vi "Vision Processing.vi"(4 "error in (no error)":errorcluster, 7 "Image Size":T1=enum."320x240") -> ()   [LabVIEW 2015]
doc: "This VI runs in parallel to other tasks. It gets images from the camera, processes them for color or shape and use that information to affect robot behavior."
uses:
  Robot Global Data.vi
  <vilib>/Rock Robotics/WPI/Camera/WPI_CameraWhite Balance Values.ctl
  <vilib>/Rock Robotics/WPI/Camera/WPI_CameraExposure Values.ctl
  <vilib>/Rock Robotics/WPI/Camera/WPI_CameraFrameRate.ctl
  <vilib>/Rock Robotics/WPI/Camera/WPI_CameraImageSize.ctl
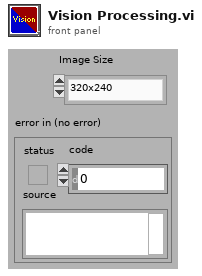
[diagram p1: front panel]
types:
  T1 = typedef "WPI_CameraImageSize.ctl" = enum16{"640x480", "320x240", "160x120"}
  T2 = typedef "WPI_CameraFrameRate.ctl" = u32
  T3 = typedef "WPI_CameraExposure Values.ctl" = enum16{"Auto", "Flicker-free 50 Hz", "Flicker-free 60 Hz", "Hold current"}
  T4 = typedef "WPI_CameraWhite Balance Values.ctl" = enum16{"Auto", "Fixed indoor", "Fixed outdoor 1", "Fixed outdoor 2", "Fixed fluorescent 1", "Fixed fluorescent 2", "Hold current"}
  T5 = typedef "Image Type" = u32
  T6 = typedef "WPI_CameraDevRef.ctl" = cluster{"Camera Address":string, "CameraStatus":errorcluster, "Acquire Image Notifier":refnum<notifier>}
  T7 = typedef "IMAQ Image.ctl" = refnum<image>
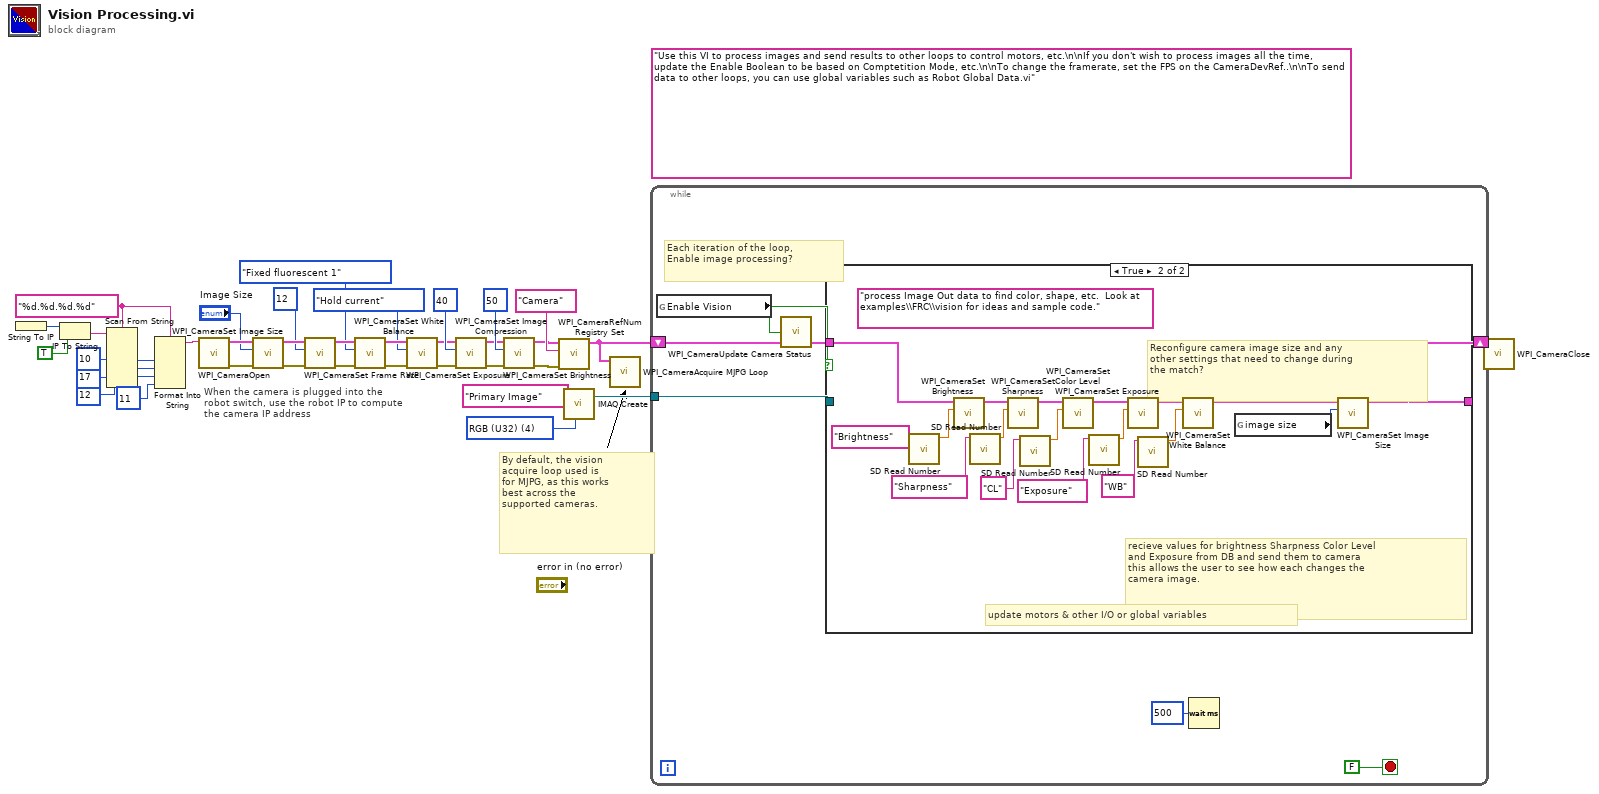
[diagram p0: block diagram]
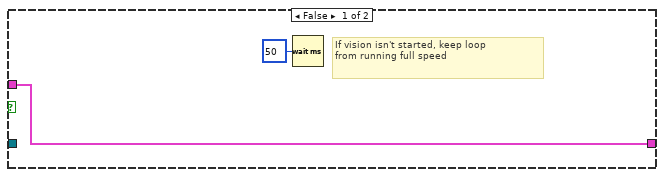
[diagram p2: hidden frame]
diagram:
  w8 = "%d.%d.%d.%d" ("format string")
  (unwired) "Use this VI to process images and send results to other loops to control motors, etc.\n\nIf you don't wish to process images all the time, update the Enable Boolean to be based on Comptetition Mode, etc.\n\nTo change the framerate, set the FPS on the CameraDevRef..\n\nTo send data to other loops, you can use global variables such as Robot Global Data.vi"
  w38 = T5 4 items=["Grayscale (U8)", "Grayscale (I16)", "Grayscale (SGL)", "Complex (CSG)", "RGB (U32)", "HSL (U32)", "RGB (U64)"] ("Image Type")
  # "When the camera is plugged into the\nrobot switch, use the robot IP to compute\nthe camera IP address"
  # "By default, the vision\nacquire loop used is\nfor MJPG, as this works\nbest across the\nsupported cameras."
  n1 = String To IP() -> (0:w15:u32)  [unwired: 1 in]
  n2 = IP To String(1:TRUE ("dot notation? (F)"), 2:w15) -> (0:w13:string)
  n3 = Scan From String(format string=w8, input string=w13, default 1=10 ("default value 1"), default 2=17 ("default value 2"), default 3=12 ("default value 3")) -> (output 1=w12:i32, output 2=w11:i32, output 3=w10:i32)  [unwired: 4 in, 3 out]
  n4 = Format Into String(format string=w8, w12, w11, w10, 11 ("Compression")) -> (resulting string=w7:string)  [unwired: 2 in, 1 out]
  n5 = call <vilib>:"WPI_CameraOpen.vi"("Camera Address"=w7) -> ("error out"=w26:errorcluster, "CameraDevRef"=w27:T6)  [unwired: 1 in, 8 out]
  n6 = call <vilib>:"WPI_CameraSet Image Size.vi"("error in (no error)"=w26, "Image Size"="Image Size", "CameraDevRef"=w27) -> ("error out"=w25:errorcluster, "CameraDevRef Out"=w28:T6)  [unwired: 7 out]
  n7 = call <vilib>:"WPI_CameraSet Frame Rate.vi"("error in (no error)"=w25, "Frame Rate (fps)"=T2 12, "CameraDevRef"=w28) -> ("error out"=w24:errorcluster, "CameraDevRef Out"=w30:T6)  [unwired: 7 out]
  n8 = call <vilib>:"WPI_CameraSet White Balance.vi"("error in (no error)"=w24, "White Balance"=WPI_CameraWhite_Balance_Values."Fixed fluorescent 1", "CameraDevRef"=w30) -> ("error out"=w23:errorcluster, "CameraDevRef Out"=w29:T6)  [unwired: 7 out]
  n9 = call <vilib>:"WPI_CameraSet Exposure.vi"("error in (no error)"=w23, "Exposure"=WPI_CameraExposure_Values."Hold current", "CameraDevRef"=w29) -> ("error out"=w22:errorcluster, "CameraDevRef Out"=w32:T6)  [unwired: 7 out]
  n10 = call <vilib>:"WPI_CameraSet Image Compression.vi"("error in (no error)"=w22, "Compression"=40, "CameraDevRef"=w32) -> ("error out"=w21:errorcluster, "CameraDevRef Out"=w31:T6)  [unwired: 7 out]
  n11 = call <vilib>:"WPI_CameraSet Brightness.vi"("error in (no error)"=w21, "Brightness"=50, "CameraDevRef"=w31) -> ("error out"=w19:errorcluster, "CameraDevRef Out"=w20:T6)  [unwired: 7 out]
  n12 = call <vilib>:"WPI_CameraRefNum Registry Set.vi"("error in (no error)"=w19, "refnum name"="Camera", "CameraDevRef"=w20) -> ("CameraDevRef"=w6:T6)  [unwired: 8 out]
  n13 = call "IMAQ Create"("Image Name"="Primary Image", "Image Type"=w38) -> ("New Image"=w36:T7)  [unwired: 2 in, 2 out]
  n14 = call <vilib>:"WPI_CameraAcquire MJPG Loop.vi"("CameraDevRef"=w6) -> ()  [unwired: 11 in]
  n15 = while {
    shift-right: [w42] -> w4
    shift-left: w6 -> [w45]
    tunnel: w36 -> [w44]
    stop <- FALSE stop-if-true
    # "Each iteration of the loop,\nEnable image processing?"
    n16 = global read "Robot Global Data.vi" "Enable Vision"() -> (w43:bool)
    n17 = call <vilib>:"WPI_CameraUpdate Camera Status.vi"("CameraDevRef In"=w45, "Enable Vision"=w43) -> ("CameraDevRef Out"=w41:T6)  [unwired: 3 in]
    n18 = case shown="True" w43 {
      tunnel: [w46 w65] -> w42
      tunnel: w44 -> [_ _]
      tunnel: w41 -> [w46 w48]
      frame False {
        # "If vision isn't started, keep loop\nfrom running full speed"
        n19 = Wait (ms)(milliseconds to wait=u32 50) -> ()  [unwired: 1 out]
      }
      frame True {
        (unwired) "process Image Out data to find color, shape, etc.  Look at examples\\FRC\\vision for ideas and sample code."
        # "recieve values for brightness Sharpness Color Level\nand Exposure from DB and send them to camera\nthis allows the user to see how each changes the \ncamera image."
        # "update motors & other I/O or global variables"
        # "Reconfigure camera image size and any\nother settings that need to change during\nthe match?"
        n20 = call <vilib>:"SD Read Number.vi"("Name"="Brightness") -> ("Numeric"=w60:dbl)  [unwired: 8 in, 2 out]
        n21 = call <vilib>:"WPI_CameraSet Brightness.vi"("Brightness"=w60, "CameraDevRef"=w48) -> ("CameraDevRef Out"=w62:T6)  [unwired: 8 in, 1 out]
        n22 = call <vilib>:"SD Read Number.vi"("Name"="Sharpness") -> ("Numeric"=w54:dbl)  [unwired: 8 in, 2 out]
        n23 = call <vilib>:"WPI_CameraSet Sharpness.vi"("Sharpness"=w54, "CameraDevRef"=w62) -> ("CameraDevRef Out"=w63:T6)  [unwired: 8 in, 1 out]
        n24 = call <vilib>:"SD Read Number.vi"("Name"="CL") -> ("Numeric"=w53:dbl)  [unwired: 8 in, 2 out]
        n25 = call <vilib>:"WPI_CameraSet Color Level.vi"("Color Level"=w53, "CameraDevRef"=w63) -> ("CameraDevRef Out"=w61:T6)  [unwired: 8 in, 1 out]
        n26 = call <vilib>:"SD Read Number.vi"("Name"="Exposure") -> ("Numeric"=w56:dbl)  [unwired: 8 in, 2 out]
        n27 = call <vilib>:"WPI_CameraSet Exposure.vi"("Exposure"=w56, "CameraDevRef"=w61) -> ("CameraDevRef Out"=w52:T6)  [unwired: 8 in, 1 out]
        n28 = call <vilib>:"SD Read Number.vi"("Name"="WB") -> ("Numeric"=w50:dbl)  [unwired: 8 in, 2 out]
        n29 = call <vilib>:"WPI_CameraSet White Balance.vi"("White Balance"=w50, "CameraDevRef"=w52) -> ("CameraDevRef Out"=w51:T6)  [unwired: 8 in, 1 out]
        n30 = global read "Robot Global Data.vi" "image size"() -> (w64:T1)
        n31 = call <vilib>:"WPI_CameraSet Image Size.vi"("Image Size"=w64, "CameraDevRef"=w51) -> ("CameraDevRef Out"=w65:T6)  [unwired: 1 in, 8 out]
      }
    }
    n32 = Wait (ms)(milliseconds to wait=u32 500) -> ()  [unwired: 1 out]
  }
  n33 = call <vilib>:"WPI_CameraClose.vi"("CameraDevRef"=w4) -> ()  [unwired: 1 in, 10 out]
